vi "Using Mask with Picture.vi"() -> ()   [LabVIEW 2016]
doc: "Masking is used when you don't want to draw certain colors of an image onto the picture control. This means that if an image has already been drawn onto the control, then masking out certain colors makes those sections of the new picture appear transparent with the original picture showing through. Multiple colors can be masked by using the combine mask option and selecting all the colors that you want to mask out."
uses:
  <vilib>/picture/picture.llb/imagedata.ctl
panel:
  in  "Image output":u16(ring) items=["Masked Picture", "Mask", "Background"]
  out "Resulting Picture":picture
  out "Color Selection":picture
  in  "Combine Masks":bool
  in  "Stop":bool
  out "Current Mask Color":u32(colorbox)
  # "Overview: Demonstrates the use of the Create Mask VI to mask one or more colors within an image.\nInstructions:\n1. Run the VI. Change the Image output to select the Mask image, which will be masked, and the background image, then change it back to Masked Picture.\n2. Click on a color within the Color Selection that you want to mask out, and watch the background picture become visible.\n3. Select Combine Masks to see the effect of combining all previous masks within the image.\n4. Click Stop to stop the VI."
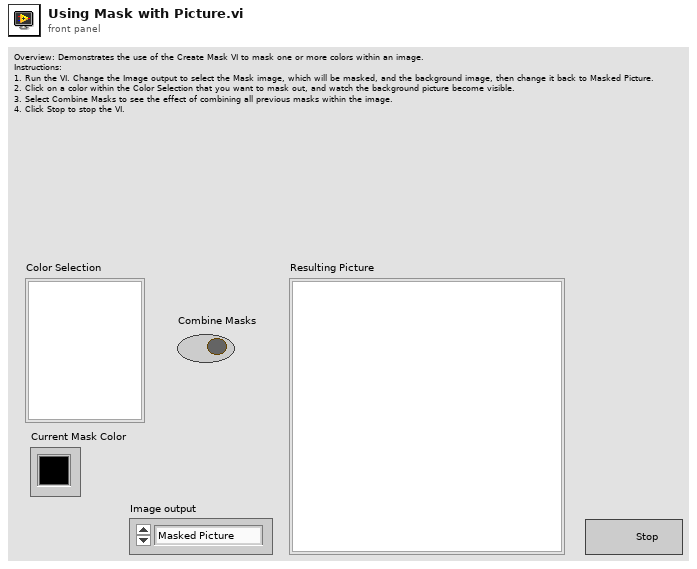
[diagram p1: front panel]
types:
  T1 = typedef "imagedata.ctl" = cluster{"image type":i32, "image depth":i32, "image":u8[], "mask":u8[], "colors":u32[], "Rectangle":cluster{"left":i16, "top":i16, "right":i16, "bottom":i16}}
  T2 = typedef "LVMouseTypeDef.ctl" = cluster{"Mouse Position":cluster{"X":i32, "Y":i32}, "Mouse Modifiers":cluster{"Button Down":bool, "Shift Mod":bool, "Menu Mod":bool, "Option Mod":bool}}
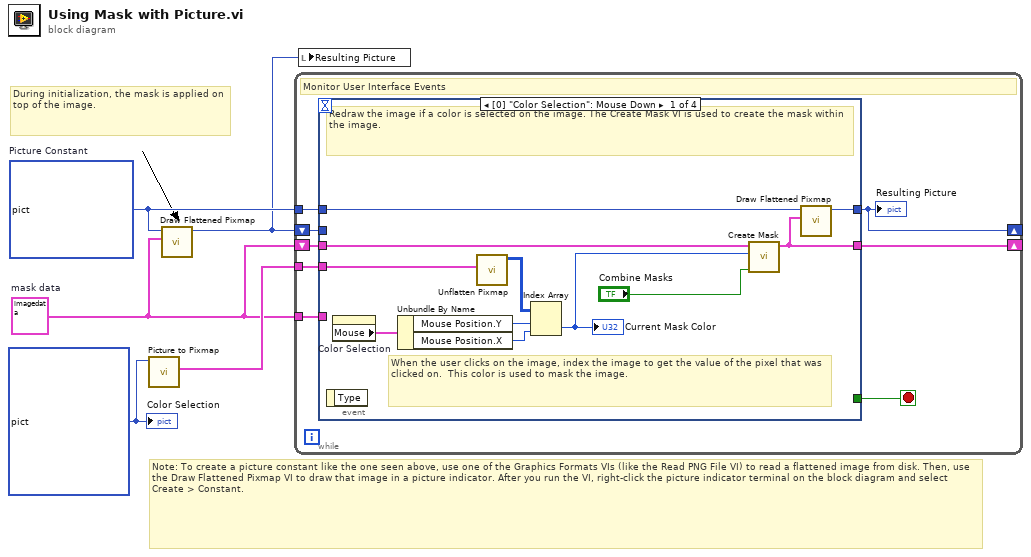
[diagram p0: block diagram]
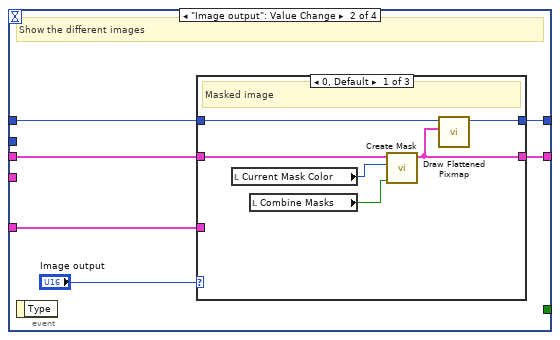
[diagram p2: hidden frame]
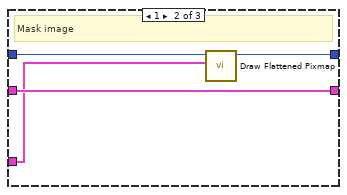
[diagram p3: hidden frame]
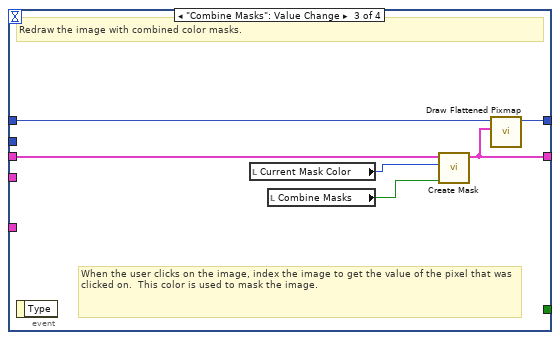
[diagram p5: hidden frame]
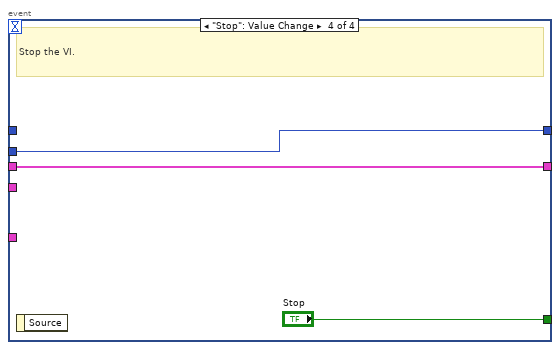
[diagram p6: hidden frame]
diagram:
  w3 = picture bytes[47088] ("Picture")
  w5 = picture bytes[255630]  # Picture Constant
  w1 = T1 {"image type"=0, "image depth"=24, "image"=array[302784 elements], "mask"=[], "colors"=[], "Rectangle"={"left"=0, "top"=0, "right"=332, "bottom"=304}}  # mask data
  # "Note: To create a picture constant like the one seen above, use one of the Graphics Formats VIs (like the Read PNG File VI) to read a flattened image from disk. Then, use the Draw Flattened Pixmap VI to draw that image in a picture indicator. After you run the VI, right-click the picture indicator terminal on the block diagram and select Create > Constant."
  # "During initialization, the mask is applied on top of the image."
  n1 = call <vilib>:"Picture to Pixmap.vi"("picture"=w3) -> ("image data"=w2:T1)  [unwired: 9 in, 1 out]
  n2 = call <vilib>:"Draw Flattened Pixmap.vi"("image data"=w1, "picture"=w5) -> ("new picture"=w4:picture)  [unwired: 7 in]
  n3 = while {
    shift-right: [w8] -> _
    shift-left: w4 -> [w11]
    tunnel: w5 -> [w12]
    shift-right: [w9] -> _
    shift-left: w1 -> [w10]
    tunnel: w2 -> [w7]
    tunnel: w1 -> [w6]
    stop <- w13 stop-if-true
    # "Monitor User Interface Events"
    n4 = event shown="[0] \"Color Selection\": Mouse Down" {
      selector: _ -> [_ _ _ _]
      dyn-events: _ -> [_ _ _ _]
      timeout: _ -> [_ _ _ _]
      tunnel: [_ _ _ "Stop"] -> w13
      tunnel: [w23 w29 w47 w50] -> w8
      tunnel: w10 -> [w14 w28 w45 w49]
      tunnel: w12 -> [w24 w30 w48 _]
      tunnel: w11 -> [_ _ _ w50]
      tunnel: [w21 w27 w46 w49] -> w9
      tunnel: w7 -> [w15 _ _ _]
      tunnel: w6 -> [_ w25 _ _]
      event "Color Selection": Mouse Down {
        # "When the user clicks on the image, index the image to get the value of the pixel that was clicked on.  This color is used to mask the image."
        # "Redraw the image if a color is selected on the image. The Create Mask VI is used to create the mask within the image."
        n5 = event-data() -> ()  [unwired: 1 in, 1 out]
        n6 = property on="Color Selection" class="Pict"() -> ("Mouse"=w18:T2)  [unwired: 2 in, 2 out]
        n7 = Unbundle By Name(w18) -> ("Mouse Position.Y"=w17:i32, "Mouse Position.X"=w16:i32)
        n8 = call <vilib>:"Unflatten Pixmap.vi"("image data"=w15) -> ("24-bit pixmap"=w22:u32[][])  [unwired: 4 in, 6 out]
        n9 = Index Array(array=w22, index (row)=w17, index (col)=w16) -> (element=w20:u32)
        "Current Mask Color" <- w20
        n10 = call <vilib>:"Create Mask.vi"("Combine Masks? (F)"="Combine Masks", "Mask Color (Black)"=w20, "image data"=w14) -> ("image data"=w21:T1)  [unwired: 8 in]
        n11 = call <vilib>:"Draw Flattened Pixmap.vi"("image data"=w21, "picture"=w24) -> ("new picture"=w23:picture)  [unwired: 7 in]
      }
      event "Image output": Value Change {
        # "Show the different images"
        n12 = event-data() -> ()  [unwired: 1 in, 1 out]
        n13 = case shown="0, Default" "Image output" {
          tunnel: [w33 w38 w42] -> w29
          tunnel: w30 -> [w34 w39 w42]
          tunnel: w28 -> [w31 w40 w41]
          tunnel: [w32 w40 w41] -> w27
          tunnel: w25 -> [_ w37 _]
          frame 0, Default {
            # "Masked image"
            n14 = local read "Current Mask Color"() -> (w35:u32)
            n15 = local read "Combine Masks"() -> (w36:bool)
            n16 = call <vilib>:"Create Mask.vi"("Combine Masks? (F)"=w36, "Mask Color (Black)"=w35, "image data"=w31) -> ("image data"=w32:T1)  [unwired: 8 in]
            n17 = call <vilib>:"Draw Flattened Pixmap.vi"("image data"=w32, "picture"=w34) -> ("new picture"=w33:picture)  [unwired: 7 in]
          }
          frame 1 {
            # "Mask image"
            n18 = call <vilib>:"Draw Flattened Pixmap.vi"("image data"=w37, "picture"=w39) -> ("new picture"=w38:picture)  [unwired: 7 in]
          }
          frame 2 {
            # "Background image"
          }
        }
      }
      event "Combine Masks": Value Change {
        # "When the user clicks on the image, index the image to get the value of the pixel that was clicked on.  This color is used to mask the image."
        # "Redraw the image with combined color masks."
        n19 = event-data() -> ()  [unwired: 1 in, 1 out]
        n20 = local read "Current Mask Color"() -> (w43:u32)
        n21 = local read "Combine Masks"() -> (w44:bool)
        n22 = call <vilib>:"Create Mask.vi"("Combine Masks? (F)"=w44, "Mask Color (Black)"=w43, "image data"=w45) -> ("image data"=w46:T1)  [unwired: 8 in]
        n23 = call <vilib>:"Draw Flattened Pixmap.vi"("image data"=w46, "picture"=w48) -> ("new picture"=w47:picture)  [unwired: 7 in]
      }
      event "Stop": Value Change {
        # "Stop the VI."
        n24 = event-data() -> ()  [unwired: 1 in, 1 out]
      }
    }
    "Resulting Picture" <- w8
  }
  n25 = local write "Resulting Picture"(w4) -> ()
  "Color Selection" <- w3
